vi "Extrinsic_transform.vi"(8 "resolution":i32[](array[numeric]), 10 "extrinsic":dbl[][](array[numeric]), 11 "X":dbl[][](array[numeric])) -> (3 "X'":dbl[][](array[numeric]))   [LabVIEW 2017]
uses:
  <vilib>/Analysis/Matrix/Numeric/Conversions/Array To Matrix - RA2.vi
  <vilib>/Analysis/Matrix/Numeric/Conversions/Matrix To Array - RM.vi
  <vilib>/Analysis/Matrix/Numeric/Multiply/Multiply - RM,RM.vi
  <vilib>/Analysis/Matrix/NI_Matrix.lvlib
panel:
  out "subarray":dbl[][](array[numeric])
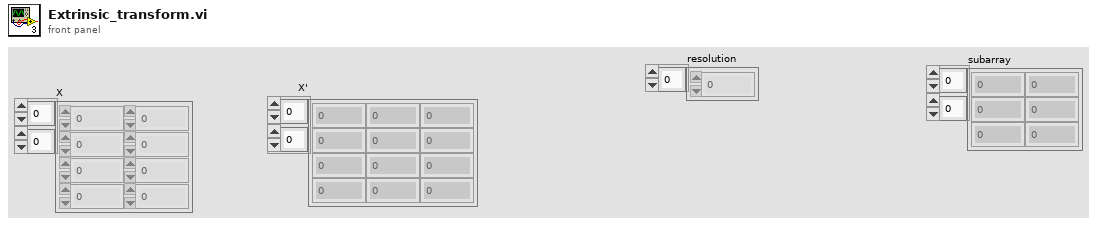
[diagram p1: front panel]
types:
  T1 = typedef "NI_Matrix.lvlib/RealMatrix.ctl" = dbl[][]
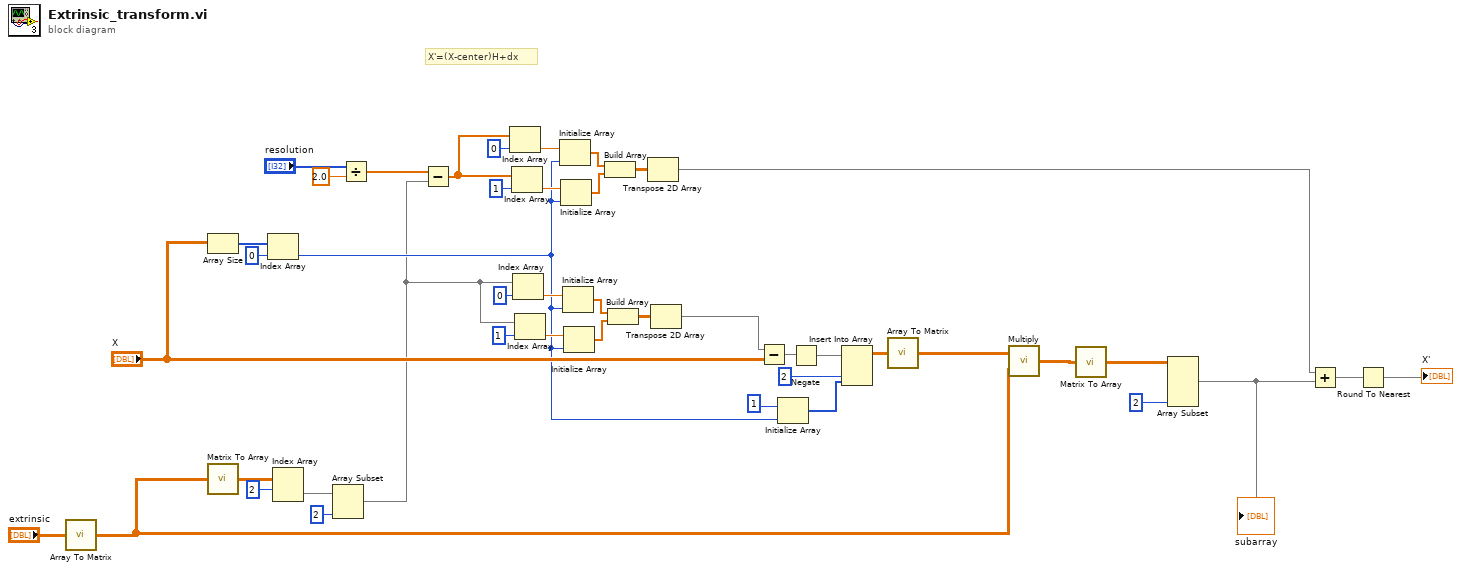
[diagram p0: block diagram]
diagram:
  # "X'=(X-center)H+dx"
  n1 = call-poly <vilib>:"Array To Matrix.vi"("Real 2D Array"="extrinsic") -> ("Real Matrix"=w34:T1)
  n2 = Array Size(array="X") -> (size(s)=w19:i32[])
  n3 = call-poly <vilib>:"Matrix To Array.vi"("Real Matrix"=w34) -> ("Real 2D Array"=w41:dbl[][])
  n4 = Index Array(array=w19, index=0) -> (element=w2:i32)
  n5 = Index Array(array=w41, index (row)=2) -> (element=w42:dbl[])  [unwired: 1 in]
  n6 = Array Subset(array=w42, length=2) -> (w1:dbl[])  [unwired: 1 in]
  n7 = Divide(x="resolution", y=2.0) -> (x/y=w27:dbl[])
  n8 = Subtract(x=w27, y=w1) -> (x-y=w26:dbl[])
  n9 = Index Array(array=w26, index=0) -> (element=w23:dbl)
  n10 = Index Array(array=w26, index=1) -> (element=w22:dbl)
  n11 = Index Array(array=w1, index=0) -> (element=w9:dbl)
  n12 = Index Array(array=w1, index=1) -> (element=w10:dbl)
  n13 = Initialize Array(w23, w2) -> (w18:dbl[])
  n14 = Initialize Array(w22, w2) -> (w17:dbl[])
  n15 = Initialize Array(w9, w2) -> (w4:dbl[])
  n16 = Initialize Array(w10, w2) -> (w3:dbl[])
  n17 = Build Array(w18, w17) -> (w16:dbl[][])
  n18 = Build Array(w4, w3) -> (w5:dbl[][])
  n19 = Transpose 2D Array(2D array=w16) -> (transposed array=w15:dbl[][])
  n20 = Transpose 2D Array(2D array=w5) -> (transposed array=w6:dbl[][])
  n21 = Subtract ("Subtract.vi")(x=w6, y="X") -> (x-y=w36:dbl[][])
  n22 = Initialize Array(1, w2) -> (w12:i32[])
  n23 = Negate(x=w36) -> (-x=w37:dbl[][])
  n24 = Insert Into Array(array=w37, index (col)=2 ("disabled index (col)"), new element=w12) -> (w38:dbl[][])  [unwired: 1 in]
  n25 = call-poly <vilib>:"Array To Matrix.vi"("Real 2D Array"=w38) -> ("Real Matrix"=w40:T1)
  n26 = call-poly <vilib>:"Multiply.vi"("Real Matrix B"=w34, "Real Matrix A"=w40) -> ("A * B"=w35:T1)
  n27 = call-poly <vilib>:"Matrix To Array.vi"("Real Matrix"=w35) -> ("Real 2D Array"=w32:dbl[][])
  n28 = Array Subset(array=w32, length (col)=2 ("length")) -> (w14:dbl[][])  [unwired: 3 in]
  "subarray" <- w14
  n29 = Add(x=w15, y=w14) -> (x+y=w13:dbl[][])
  n30 = Round To Nearest(number=w13) -> (nearest integer value=→"X'":dbl[][])
